vi "QueueTester.vi"() -> ()   [LabVIEW 2013]
panel:
  out "Queue Size":i32
  in  "Dequeue":bool
  in  "Enqueue":bool
  in  "element":enum16{"A", "B", "C", "D"}(ring)
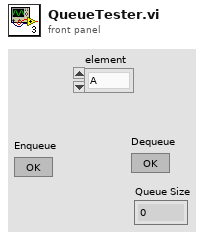
[diagram p1: front panel]
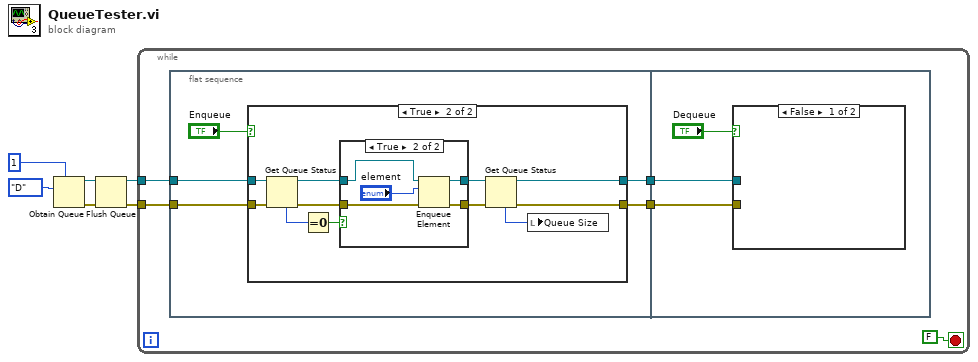
[diagram p0: block diagram]
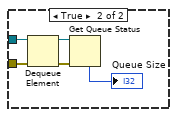
[diagram p4: hidden frame]
diagram:
  n1 = Obtain Queue(max queue size (-1, unlimited)=1, element data type=enum16{"A", "B", "C", "D"}."D") -> (queue out=w4:refnum<queue>, error out=w5:errorcluster)  [unwired: 3 in, 1 out]
  n2 = Flush Queue(queue=w4, error in (no error)=w5) -> (queue out=w3:refnum<queue>, error out=w2:errorcluster)  [unwired: 1 out]
  n3 = while {
    tunnel: w3 -> [w11]
    tunnel: w2 -> [w10]
    stop <- FALSE stop-if-true
    n4 = flat-sequence {
      tunnel: w11 -> [w16]
      tunnel: w10 -> [w15]
      tunnel: [w13] -> w8
      tunnel: [w12] -> w7
      tunnel: w8 -> [w38]
      tunnel: w7 -> [w37]
      frame #0 {
        n5 = case shown="True" "Enqueue" {
          tunnel: w16 -> [w17 w25]
          tunnel: w15 -> [w18 w24]
          tunnel: [w17 w27] -> w13
          tunnel: [w18 w26] -> w12
          frame False {
          }
          frame True {
            n6 = Get Queue Status(queue=w25, error in (no error)=w24) -> (queue out=w23:refnum<queue>, error out=w22:errorcluster, # elements in queue=w20:i32)  [unwired: 1 in, 5 out]
            n7 = Equal To 0?(x=w20) -> (x = 0?=w21:bool)
            n8 = case shown="True" w21 {
              tunnel: [w31 w35] -> w29
              tunnel: [w30 w34] -> w28
              tunnel: w23 -> [w31 w33]
              tunnel: w22 -> [w30 w32]
              frame False {
              }
              frame True {
                n9 = Enqueue Element(queue=w33, element="element", error in (no error)=w32) -> (queue out=w35:refnum<queue>, error out=w34:errorcluster)  [unwired: 1 in, 1 out]
              }
            }
            n10 = Get Queue Status(queue=w29, error in (no error)=w28) -> (queue out=w27:refnum<queue>, error out=w26:errorcluster, # elements in queue=w19:i32)  [unwired: 1 in, 5 out]
            n11 = local write "Queue Size"(w19) -> ()
          }
        }
      }
      frame #1 {
        n12 = case shown="False" "Dequeue" {
          tunnel: w38 -> [_ w41]
          tunnel: w37 -> [_ w40]
          frame False {
          }
          frame True {
            n13 = Dequeue Element(queue=w41, error in (no error)=w40) -> (queue out=w44:refnum<queue>, error out=w43:errorcluster)  [unwired: 1 in, 2 out]
            n14 = Get Queue Status(queue=w44, error in (no error)=w43) -> (# elements in queue=→"Queue Size":i32)  [unwired: 1 in, 7 out]
          }
        }
      }
    }
  }
